vi "OAT Order Magnitude and Phase Plot(XY).vi"   [LabVIEW 2017, in "SoundVib_Resampling.lvlib"]
uses:
  <vilib>/addons/Sound and Vibration/Order Analysis/Resample Order Tracking/SoundVib_Resampling.lvlib
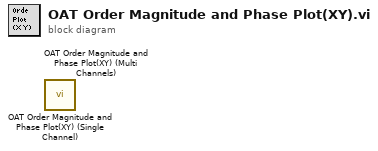
[diagram p0: block diagram]
diagram:
  n1 = call <vilib>:"OAT Order Magnitude and Phase Plot(XY) (Single Channel).vi"() -> ()  [unwired: 9 in, 3 out]
  n2 = call <vilib>:"OAT Order Magnitude and Phase Plot(XY) (Multi Channels).vi"() -> ()  [unwired: 9 in, 3 out]
